vi "Body(SubVI).vi"(3 "error in":errorcluster caption="error in\nerror in", 4 "문자열":string, 5 "VISA resource name out 2":refnum<visa-resource-name>) -> (0 "error out":errorcluster, 1 "read buffer":string, 2 "VISA resource name out":refnum<visa-resource-name>)   [LabVIEW 2010]
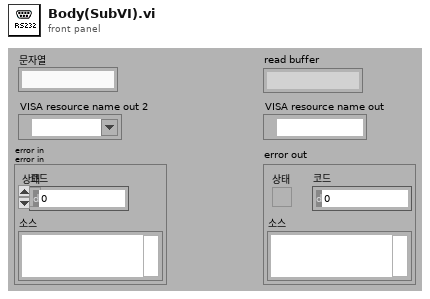
[diagram p1: front panel]
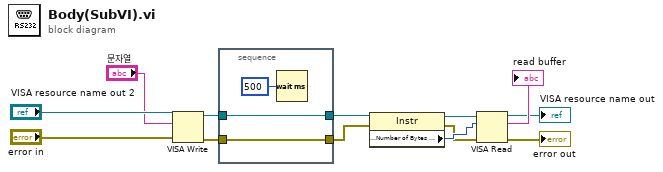
[diagram p0: block diagram]
diagram:
  n1 = VISA Write(VISA resource name="VISA resource name out 2", write buffer="문자열", error in (no error)="error in") -> (VISA resource name out=w4:refnum<visa-resource-name>, error out=w5:errorcluster)  [unwired: 1 out]
  n2 = stacked-sequence {
    tunnel: w4 -> [w16]
    tunnel: w5 -> [w15]
    tunnel: [w16] -> w6
    tunnel: [w15] -> w7
    frame #0 {
      n3 = Wait (ms)(milliseconds to wait=u32 500 ("기다릴 ms")) -> ()  [unwired: 1 out]
    }
  }
  n4 = property class="Instr"(reference=w6, error in=w7) -> (reference out=w8:refnum<visa-resource-name>, error out=w9:errorcluster, "Serial Settings:Number of Bytes at Serial Port"=w12:u32)
  n5 = VISA Read(VISA resource name=w8, byte count=w12, error in (no error)=w9) -> (VISA resource name out=→"VISA resource name out":refnum<visa-resource-name>, read buffer=→"read buffer":string, error out=→"error out":errorcluster)  [unwired: 1 out]
